vi "PCO_GetAcquireModeEx.vi"(8 "error in (no error)":errorcluster {"code" format="%x"}, 11 "ph":u64) -> (0 "error out":errorcluster {"code" format="%x"}, 1 "wAcquMode":u16(ring) items=["auto", "external", "external modulate", "", "sequence trigger"], 2 "ErrorMessage":i32 format="%x", 3 "ph out":u64, 5 "dwNumberImages":u32)   [LabVIEW 2019, in "SDK.lvlib" / "RecordingControl.lvlib"]
doc: "<b>Description:</b>\nThis function returns the current acquire mode of the camera. Acquire mode can be either [auto], [external], [external modulate] or [sequence trigger].\nThis function is an extended version of the PCO_GetAcquireMode function with an additional parameter dwNumberImages, which is needed for the [sequence trigger] mode.\n\n<b>Supported camera type:</b>\npco.edge\n\n<b>Descriptor dependency:</b>\ndwGeneralCapsDESC1: NO_ACQUIREMODE,EXT_ACQUIRE"
uses:
  RecordingControl.lvlib
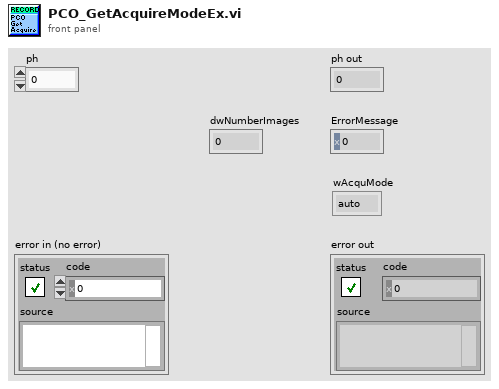
[diagram p1: front panel]
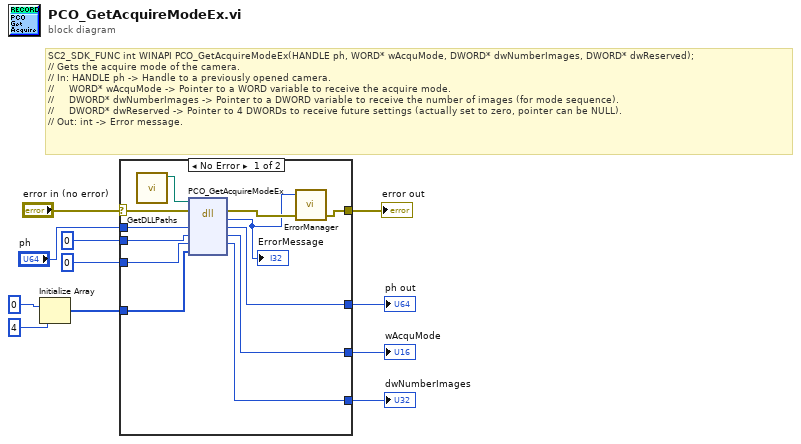
[diagram p0: block diagram]
diagram:
  # "SC2_SDK_FUNC int WINAPI PCO_GetAcquireModeEx(HANDLE ph, WORD* wAcquMode, DWORD* dwNumberImages, DWORD* dwReserved);\n// Gets the acquire mode of the camera.\n// In: HANDLE ph -> Handle to a previously opened camera.\n//     WORD* wAcquMode -> Pointer to a WORD variable to receive the acquire mode.\n//     DWORD* dwNumberImages -> Pointer to a DWORD variable to receive the number of images (for mode sequence).\n//     DWORD* dwReserved -> Pointer to 4 DWORDs to receive future settings (actually set to zero, pointer can be NULL).\n// Out: int -> Error message."
  n1 = Initialize Array(u32 0 ("dwReserved"), 4 ("dimension size")) -> (w1:u32[])
  n2 = case shown="No Error" "error in (no error)" {
    selector: "error in (no error)" -> [w16 w27]
    tunnel: "ph" -> [w23 w26]
    tunnel: [w22 w26] -> w10
    tunnel: u16 0 ("wAcquMode") -> [w21 w25]
    tunnel: [w20 w25] -> w8
    tunnel: u32 0 ("dwNumberImages") -> [w19 w24]
    tunnel: [w18 w24] -> w6
    tunnel: w1 -> [w17 _]
    tunnel: [w14 w27] -> w5
    frame No Error {
      n3 = call "GetDLLPaths.vi"() -> ("SC2_Cam_Path"=w12:path)  [unwired: 8 in, 3 out]
      n4 = dll-call lib="?" fn="PCO_GetAcquireModeEx"(path in=w12, error in=w16, "ph"=w23, "wAcquMode"=w21, "dwNumberImages"=w19, "dwReserved"=w17) -> (error out=w15:errorcluster, "return type"=w13:i32, "ph"=w22:u64, "wAcquMode"=w20:u16, "dwNumberImages"=w18:u32)  [unwired: 2 in, 1 out]
      "ErrorMessage" <- w13
      n5 = call "ErrorManager.vi"("error in (no error)"=w15, "error code"=w13) -> ("error out"=w14:errorcluster)  [unwired: 2 in, 1 out]
    }
    frame Error {
    }
  }
  "ph out" <- w10
  "wAcquMode" <- w8
  "dwNumberImages" <- w6
  "error out" <- w5
